vi "Configure Reference Power.vi"(6 "Fine Scale Adjust (0)":u16, 7 "Coarse Scale Adjust (0)":u16, 8 "error in (no error)":errorcluster, 9 "Adjust Output Power (F: Disable)":bool, 10 "Enable Reference Power (F: Disable)":bool, 11 "VISA resource name":refnum<visa-resource-name>) -> (0 "error out":errorcluster, 3 "VISA resource name out":refnum<visa-resource-name>)   [LabVIEW 2011, in "Agilent N432A.lvlib"]
doc: "Enables the Reference Power and adjusts the value of output."
uses:
  <instrlib>/Agilent N432A/Agilent N432A.lvlib
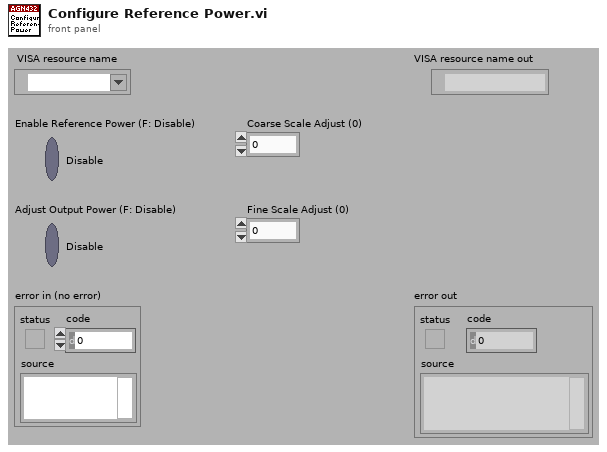
[diagram p1: front panel]
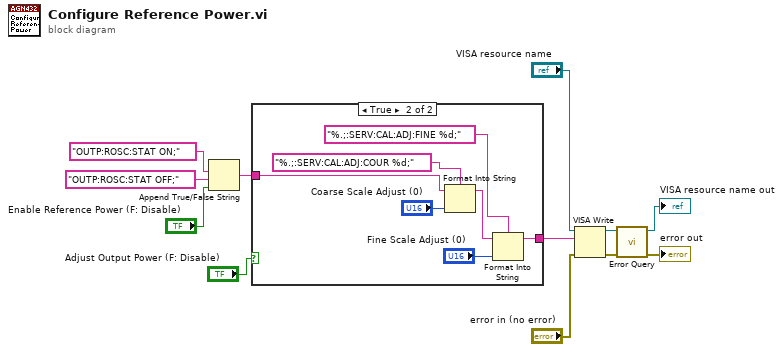
[diagram p0: block diagram]
diagram:
  n1 = Append True/False String(1:"Enable Reference Power (F: Disable)", 2:"OUTP:ROSC:STAT OFF;", 3:"OUTP:ROSC:STAT ON;") -> (0:w9:string)  [unwired: 1 in]
  n2 = case shown="True" "Adjust Output Power (F: Disable)" {
    tunnel: w9 -> [w13 w20]
    tunnel: [w13 w14] -> w8
    frame False {
    }
    frame True {
      n3 = Format Into String(format string="%.;:SERV:CAL:ADJ:COUR %d;", initial string=w20, "Coarse Scale Adjust (0)") -> (resulting string=w17:string)  [unwired: 1 in, 1 out]
      n4 = Format Into String(format string="%.;:SERV:CAL:ADJ:FINE %d;", initial string=w17, "Fine Scale Adjust (0)") -> (resulting string=w14:string)  [unwired: 1 in, 1 out]
    }
  }
  n5 = VISA Write(VISA resource name="VISA resource name", write buffer=w8, error in (no error)="error in (no error)") -> (VISA resource name out=w5:refnum<visa-resource-name>, error out=w4:errorcluster)  [unwired: 1 out]
  n6 = call <instrlib>:"Error Query.vi"("error in (no error)"=w4, "VISA resource name"=w5) -> ("error out"=→"error out":errorcluster, "VISA resource name out"=→"VISA resource name out":refnum<visa-resource-name>)  [unwired: 6 in, 2 out]
